vi "Setting_BK9201.vi"(0 "Instrument In":refnum<visa-resource-name>, 2 "Set Out Voltage":dbl format="%.3g", 3 "Current Limit":dbl min=0.0 max=25.0 step=1.0 format="%.4f", 4 "Over Voltage Limit":dbl=61.0 min=0.0 max=151.0 step=0.001 format="%.3f", 5 "error in (no error)":errorcluster, 6 "Ring":u16(ring) items=["Disable", "Enable"]) -> (14 "Instrument Out":refnum<visa-resource-name>, 19 "error out":errorcluster)   [LabVIEW 2023]
uses:
  <instrlib>/BK Precision 9200 Series/BK Precision 9200 Series.lvlib
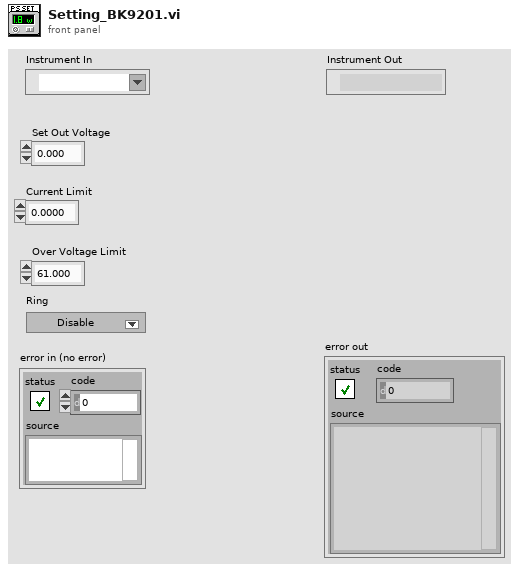
[diagram p1: front panel]
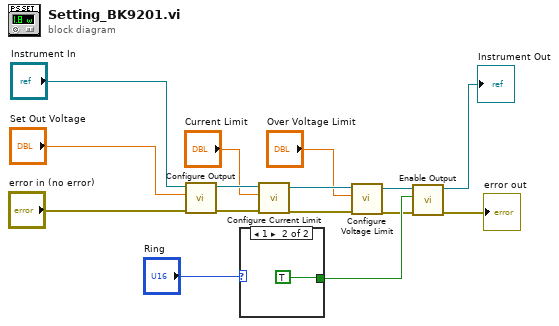
[diagram p0: block diagram]
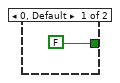
[diagram p2: hidden frame]
diagram:
  n1 = call <instrlib>:"Configure Output.vi"("error in (no error)"="error in (no error)", "Voltage Level (0.0 V)"="Set Out Voltage", "VISA resource name"="Instrument In") -> ("error out"=w11:errorcluster, "VISA resource name out"=w12:refnum<visa-resource-name>)  [unwired: 7 in]
  n2 = case shown="1" "Ring" {
    tunnel: [FALSE TRUE] -> w5
    frame 0, Default {
    }
    frame 1 {
    }
  }
  n3 = call <instrlib>:"Configure Current Limit.vi"("error in (no error)"=w11, "Current Limit (0.0 A)"="Current Limit", "VISA resource name"=w12) -> ("error out"=w8:errorcluster, "VISA resource name out"=w9:refnum<visa-resource-name>)  [unwired: 7 in]
  n4 = call <instrlib>:"Configure Voltage Limit.vi"("error in (no error)"=w8, "Max Voltage Limit (61.000 V)"="Over Voltage Limit", "VISA resource name"=w9) -> ("error out"=w4:errorcluster, "VISA resource name out"=w3:refnum<visa-resource-name>)  [unwired: 7 in]
  n5 = call <instrlib>:"Enable Output.vi"("error in (no error)"=w4, "Enable Output (F: False)"=w5, "VISA resource name"=w3) -> ("error out"=→"error out":errorcluster, "VISA resource name out"=→"Instrument Out":refnum<visa-resource-name>)  [unwired: 7 in]
